vi "CCM-Save Tables.vi"(0 "configuration file path":path=path "C:/PXI Connections.txt", 5 "Tables":cluster{"Table":T1[]}[](array[cluster]), 9 "Endpoints":cluster{"Items":string[]}[](array[cluster]), 11 "error in (no error)":errorcluster) -> (4 "file path":path, 15 "error out":errorcluster)   [LabVIEW 2020]
uses:
  Type Defs/CM-Connection.ctl
  Type Defs/CM-IO Type.ctl
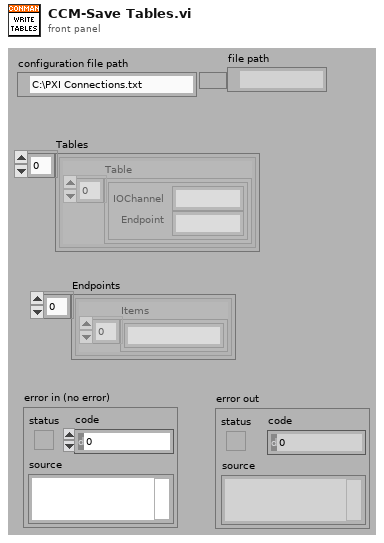
[diagram p1: front panel]
types:
  T1 = typedef "CM-Connection.ctl" = cluster{"IOChannel":string, "Endpoint":string}
  T2 = typedef "CM-IO Type.ctl" = enum16{"Analog Outputs", "Analog Inputs", "Digital Outputs", "Digital Inputs"}
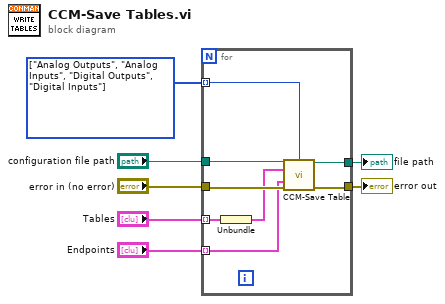
[diagram p0: block diagram]
diagram:
  w6 = T2[] [enum."Analog Outputs", enum."Analog Inputs", enum."Digital Outputs", enum."Digital Inputs"] items=["Analog Outputs", "Analog Inputs", "Digital Outputs", "Digital Inputs"]
  n1 = for {
    tunnel: [w9] -> w5
    tunnel: w6 -> [w14] mode=indexing
    tunnel: "error in (no error)" -> [w13]
    tunnel: "Endpoints" -> [w11] mode=indexing
    tunnel: "Tables" -> [w12] mode=indexing
    tunnel: "configuration file path" -> [w15]
    tunnel: [w8] -> w1
    n2 = Unbundle(w12) -> ("Table"=w10:T1[])
    n3 = call "CCM-Save Table.vi"("configuration file path"=w15, "IO Type"=w14, "Table"=w10, "Endpoints"=w11, "error in (no error)"=w13) -> ("file path"=w8:path, "error out"=w9:errorcluster)  [unwired: 9 in]
  }
  "error out" <- w5
  "file path" <- w1
